vi "Test Helper Loop Broadcast Stopped on Error.vi"(8 "error in (no error)":errorcluster, 11 "Helper Loop Test In":refnum<class "Helper Loop Test.lvclass">) -> (0 "error out":errorcluster, 3 "Helper Loop Test Out":refnum<class "Helper Loop Test.lvclass">)   [LabVIEW 2020, in "Helper Loop Test.lvclass"]
uses:
  Helper Loop Test.lvclass
  C:/Program Files (x86)/National Instruments/LabVIEW 2020/vi.lib/Asteme/LUnit/Test Case.lvclass
  Mock Process/Mock Process.lvclass
  C:/Users/anton/Documents/GitHub/Triarc-Framework/source/Framework/Process/Process.lvclass
  <vilib>/Asteme/LUnit/Test Case.lvclass/Test Case.ctl
  <vilib>/Asteme/LUnit/LUnit Assertion Result.lvclass/LUnit Assertion Result.ctl
  Framework/Process/Process.lvclass/Process.ctl
  Framework/Broadcast Event Helpers/Execution timer.vi
  <vilib>/Asteme/LUnit/Palette/Pass.vi
  <vilib>/Asteme/LUnit/Palette/Fail.vi
  <vilib>/Asteme/LUnit/Variant to string.vi
  <vilib>/Asteme/LUnit/Set Assertion Type.vi
  <vilib>/Asteme/LUnit/Palette/Pass If.vi
  Framework/Process/Private/SubVIs/Wait for finish.vi
  Framework/Process/Protected/Messaging/Enqueue Message.vi
  Framework/Process/Private/SubVIs/Set Lifecycle State.vi
  Framework/Process/Public/Lifecycle/Get Lifecycle State.vi
  <vilib>/Asteme/LUnit/Add test result.vi
  <vilib>/Asteme/LUnit/LUnit Write Passed.vi
  <vilib>/Asteme/LUnit/LUnit Get Test Case.vi
  <vilib>/Asteme/LUnit/Assertion Result/LUnit Get Test Name.vi
  <vilib>/Asteme/LUnit/LUnit Write Message.vi
  <vilib>/Asteme/LUnit/LUnit Write Description.vi
  <vilib>/Asteme/LUnit/LUnit Write Assertion Type.vi
  <vilib>/Utility/error.llb/Clear Errors.vi
  <vilib>/Asteme/LUnit/Read Test Case Name.vi
  Framework/Broadcast Event Helpers/Dequeue Broadcast Message.vi
  <vilib>/Utility/Data Type/Get Type Information.vi
  <vilib>/Utility/LVClass/Get LV Class Name.vi
  <vilib>/Utility/error.llb/Error Cluster From Error Code.vi
  <vilib>/Asteme/LUnit/LUnit Assertion Result.lvclass
  Framework/Process/Process.lvclass
  <vilib>/Asteme/LUnit/Test Case.lvclass
  Framework/Broadcast Event Helpers/Broadcast Event Helpers.lvlib
panel:
  out "timed out?":bool
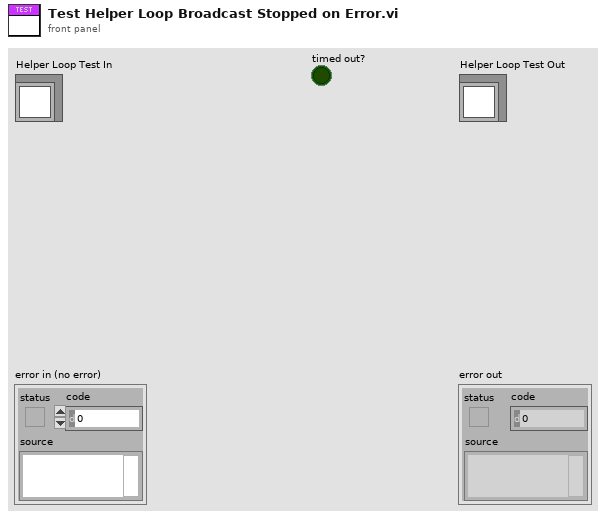
[diagram p1: front panel]
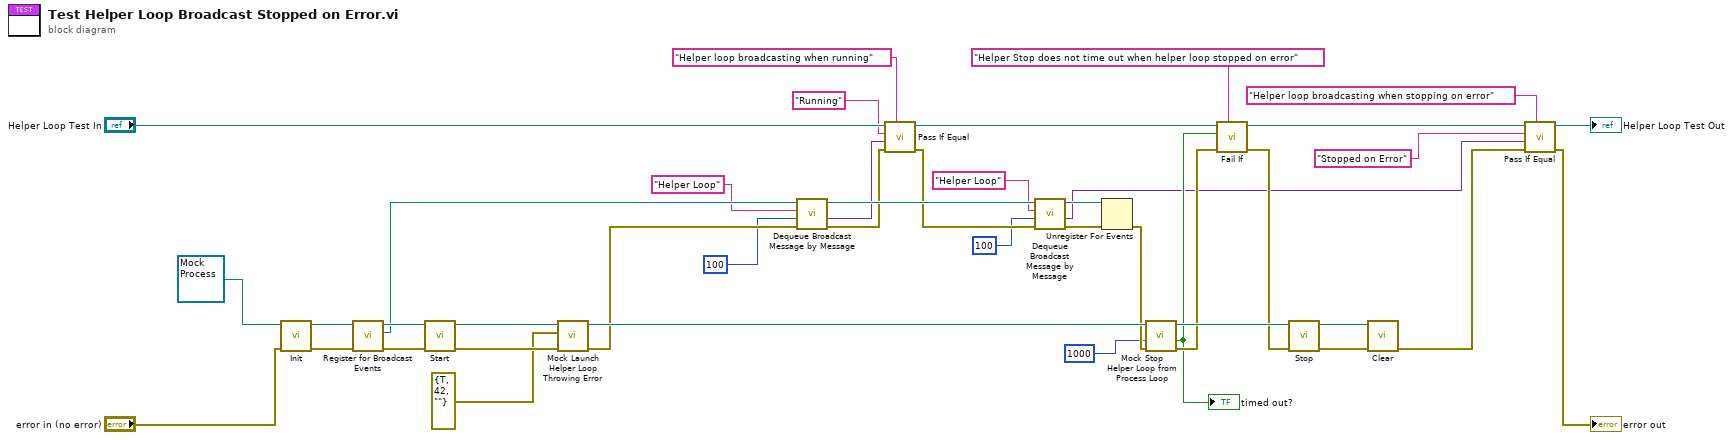
[diagram p0: block diagram]
diagram:
  n1 = call-dynamic "Init.vi"("error in (no error)"="error in (no error)", "Mock Process In"=refnum<class "Mock Process.lvclass"> refnum) -> ("error out"=w41:errorcluster, "Mock Process Out"=w42:refnum<class "Mock Process.lvclass">)  [unwired: 8 in]
  n2 = call "Register for Broadcast Events.vi"("error in (no error)"=w41, "Process In"=w42) -> ("error out"=w39:errorcluster, "Event Registration Refnum Out"=w26:refnum<event-registration>, "Process Out"=w40:refnum<class "Mock Process.lvclass">)  [unwired: 7 in]
  n3 = call "Start.vi"("error in (no error)"=w39, "Process In"=w40) -> ("error out"=w37:errorcluster, "Process Out"=w38:refnum<class "Mock Process.lvclass">)  [unwired: 8 in]
  n4 = call "Mock Launch Helper Loop Throwing Error.vi"("error in (no error)"=w37, "Error message"=errorcluster {"status"=TRUE, "code"=42, "source"=""}, "Mock Process in"=w38) -> ("error out"=w24:errorcluster, "Mock Process out"=w36:refnum<class "Mock Process.lvclass">)  [unwired: 7 in]
  n5 = call "Dequeue Broadcast Message by Message.vi"("error in (no error)"=w24, "Timeout (-1)"=100, "Message"="Helper Loop" ("y"), "Event Registration Refnum"=w26) -> ("error out"=w8:errorcluster, "Message Data"=w9:variant, "Event Registration Refnum Out"=w18:refnum<event-registration>)  [unwired: 3 in, 2 out]
  n6 = call <vilib>:"Pass If Equal.vi"("Description"="Helper loop broadcasting when running", "error in (no error)"=w8, "Actual"=w9, "Expected"="Running" ("Description"), "Test Case In"="Helper Loop Test In") -> ("error out"=w16:errorcluster, "Test Case Out"=w13:refnum<class "Helper Loop Test.lvclass">)  [unwired: 5 in]
  n7 = call "Dequeue Broadcast Message by Message.vi"("error in (no error)"=w16, "Timeout (-1)"=100, "Message"="Helper Loop" ("y"), "Event Registration Refnum"=w18) -> ("error out"=w5:errorcluster, "Message Data"=w4:variant, "Event Registration Refnum Out"=w17:refnum<event-registration>)  [unwired: 3 in, 2 out]
  n8 = Unregister For Events(event registration refnum=w17, error in=w5) -> (error out=w23:errorcluster)
  n9 = call "Mock Stop Helper Loop from Process Loop.vi"("error in (no error)"=w23, "timeout in ms (-1)"=1000, "Mock Process in"=w36) -> ("error out"=w34:errorcluster, "timed out?"=w10:bool, "Mock Process out"=w35:refnum<class "Mock Process.lvclass">)  [unwired: 6 in]
  "timed out?" <- w10
  n10 = call <vilib>:"Fail If.vi"("Description"="Helper Stop does not time out when helper loop stopped on error", "error in (no error)"=w34, "Fail?"=w10, "Test Case In"=w13) -> ("error out"=w14:errorcluster, "Test Case Out"=w12:refnum<class "Helper Loop Test.lvclass">)  [unwired: 6 in]
  n11 = call "Stop.vi"("error in (no error)"=w14, "Process In"=w35) -> ("error out"=w33:errorcluster, "Process Out"=w1:refnum<class "Mock Process.lvclass">)  [unwired: 7 in, 1 out]
  n12 = call-dynamic "Clear.vi"("error in (no error)"=w33, "Mock Process In"=w1) -> ("error out"=w32:errorcluster)  [unwired: 9 in]
  n13 = call <vilib>:"Pass If Equal.vi"("Description"="Helper loop broadcasting when stopping on error", "error in (no error)"=w32, "Actual"=w4, "Expected"="Stopped on Error" ("Description"), "Test Case In"=w12) -> ("error out"=→"error out":errorcluster, "Test Case Out"=→"Helper Loop Test Out":refnum<class "Helper Loop Test.lvclass">)  [unwired: 5 in]
